vi "get_test_log_files.vi"(8 "error in (no error)":errorcluster, 11 "params in":T1) -> (0 "error out":errorcluster, 3 "Data":T2)   [LabVIEW 2015]
doc: "This vi does the following tasks: \n1.- Create the Test Log folder and subfolders, \n2.- Get the timeout values from config file, \n3.- Get the endpoint address from config file,\n4.- Get the file extension to search (i.e *json) from config file.,\n5.- Get holding time from config file."
uses:
  Type Definitions/get_test_log_files_data.ctl
  <vilib>/Utility/error.llb/Error Cluster From Error Code.vi
  <vilib>/ErrorRing/Error Ring.xnode
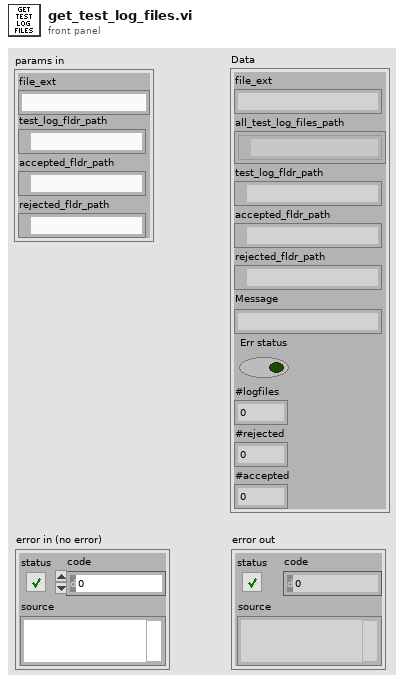
[diagram p1: front panel]
types:
  T1 = cluster{"file_ext":string, "test_log_fldr_path":path, "accepted_fldr_path":path, "rejected_fldr_path":path}
  T2 = typedef "get_test_log_files_data.ctl" = cluster{"file_ext":string, "all_test_log_files_path":path[], "test_log_fldr_path":path, "accepted_fldr_path":path, "rejected_fldr_path":path, "Message":string, "Err status":bool, "#logfiles":i32, "#rejected":i32, "#accepted":i32}
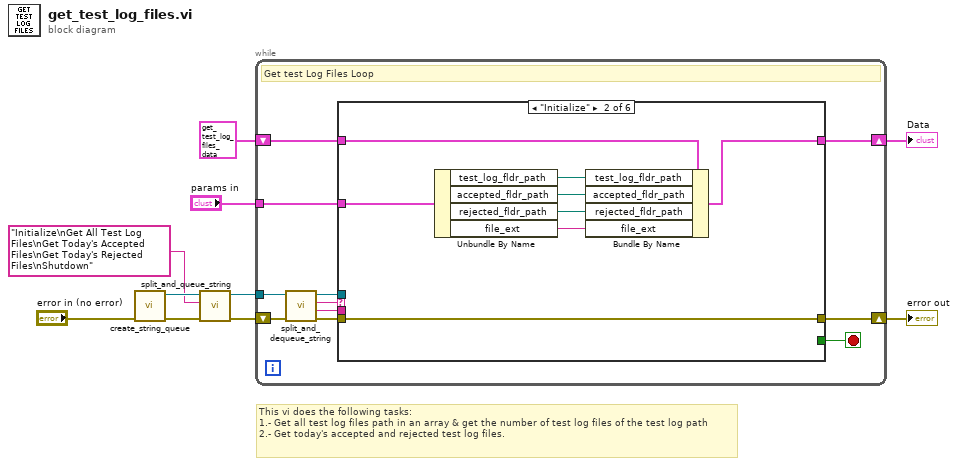
[diagram p0: block diagram]
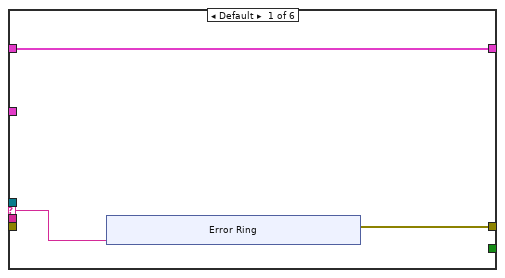
[diagram p2: hidden frame]
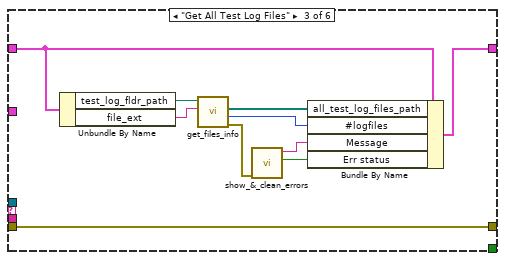
[diagram p3: hidden frame]
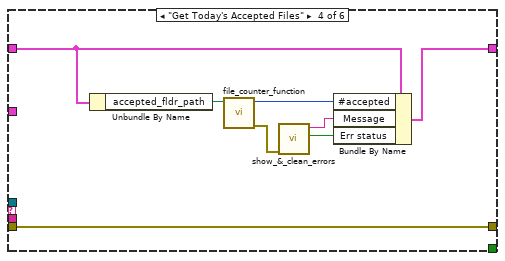
[diagram p4: hidden frame]
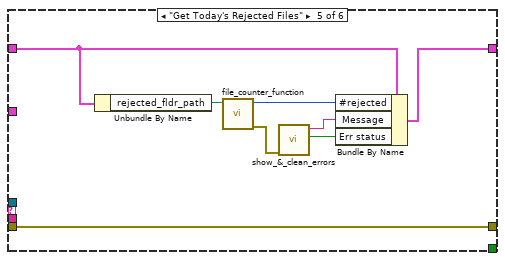
[diagram p5: hidden frame]
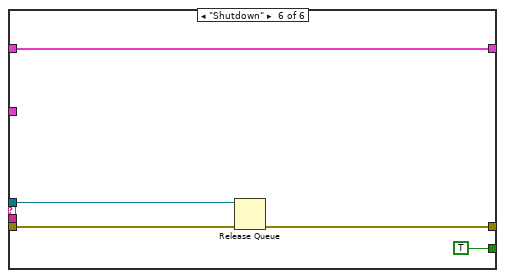
[diagram p6: hidden frame]
diagram:
  # "This vi does the following tasks:\n1.- Get all test log files path in an array & get the number of test log files of the test log path\n2.- Get today's accepted and rejected test log files."
  n1 = call "create_string_queue.vi"("error in (no error)"="error in (no error)") -> ("error out"=w9:errorcluster, "Queue out"=w10:refnum<queue>)  [unwired: 9 in]
  n2 = call "split_and_queue_string.vi"("error in (no error)"=w9, "list state:argument"="Initialize\nGet All Test Log Files\nGet Today's Accepted Files\nGet Today's Rejected Files\nShutdown", "Queue in"=w10) -> ("error out"=w8:errorcluster, "Queue out"=w7:refnum<queue>)  [unwired: 7 in]
  n3 = while {
    shift-right: [w19] -> w5
    shift-left: w8 -> [w21]
    tunnel: w7 -> [w17]
    shift-right: [w13] -> w2
    shift-left: T2 {"file_ext"="", "all_test_log_files_path"=[], "test_log_fldr_path"=path "", "accepted_fldr_path"=path "", "rejected_fldr_path"=path "", "Message"="", "Err status"=FALSE, "#logfiles"=0, "#rejected"=0, "#accepted"=0} ("Data") -> [w14]
    tunnel: "params in" -> [w11]
    stop <- w18 stop-if-true
    # "Get test Log Files Loop"
    n4 = call "split_and_dequeue_string.vi"("error in (no error)"=w21, "Queue in"=w17) -> ("error out"=w20:errorcluster, "argument"=w15:string, "state"=w16:string, "Queue out"=w12:refnum<queue>)  [unwired: 6 in]
    n5 = case shown="\"Initialize\"" w16 {
      selector: w16 -> [w23 _ _ _ _ _]
      tunnel: w20 -> [_ w39 w49 w57 w65 w69]
      tunnel: [w22 w39 w49 w57 w65 w67] -> w19
      tunnel: [_ _ _ _ _ TRUE] -> w18
      tunnel: w12 -> [_ _ _ _ _ w68]
      tunnel: w15 -> [_ _ _ _ _ _]
      tunnel: w14 -> [w24 w38 w41 w51 w59 w66]
      tunnel: [w24 w37 w40 w50 w58 w66] -> w13
      tunnel: w11 -> [_ w36 _ _ _ _]
      frame Default {
        n6 = xnode "Error Ring"("parameter 0"=w23) -> ("error out"=w22:errorcluster)
      }
      frame "Initialize" {
        n7 = Unbundle By Name(w36) -> ("test_log_fldr_path"=w34:path, "accepted_fldr_path"=w33:path, "rejected_fldr_path"=w32:path, "file_ext"=w35:string)
        n8 = Bundle By Name(cluster=w38, "test_log_fldr_path"=w34, "accepted_fldr_path"=w33, "rejected_fldr_path"=w32, "file_ext"=w35) -> (w37:T2)
      }
      frame "Get All Test Log Files" {
        n9 = Unbundle By Name(w41) -> ("test_log_fldr_path"=w47:path, "file_ext"=w48:string)
        n10 = call "get_files_info.vi"("file extension"=w48, "test_log_base_path"=w47) -> ("error out"=w42:errorcluster, "logfiles#"=w44:i32, "All files in folder"=w43:path[])  [unwired: 6 in, 1 out]
        n11 = call "show_&_clean_errors.vi"("error in (no error)"=w42) -> ("status"=w46:bool, "message out"=w45:string)  [unwired: 7 in, 2 out]
        n12 = Bundle By Name(cluster=w41, "all_test_log_files_path"=w43, "#logfiles"=w44, "Message"=w45, "Err status"=w46) -> (w40:T2)
      }
      frame "Get Today's Accepted Files" {
        n13 = Unbundle By Name(w51) -> ("accepted_fldr_path"=w54:path)
        n14 = call "file_counter_function.vi"("files_folder_path"=w54) -> ("error out"=w56:errorcluster, "#files_found"=w55:i32)  [unwired: 8 in, 1 out]
        n15 = call "show_&_clean_errors.vi"("error in (no error)"=w56) -> ("status"=w52:bool, "message out"=w53:string)  [unwired: 7 in, 2 out]
        n16 = Bundle By Name(cluster=w51, "#accepted"=w55, "Message"=w53, "Err status"=w52) -> (w50:T2)
      }
      frame "Get Today's Rejected Files" {
        n17 = Unbundle By Name(w59) -> ("rejected_fldr_path"=w62:path)
        n18 = call "file_counter_function.vi"("files_folder_path"=w62) -> ("error out"=w64:errorcluster, "#files_found"=w63:i32)  [unwired: 8 in, 1 out]
        n19 = call "show_&_clean_errors.vi"("error in (no error)"=w64) -> ("status"=w60:bool, "message out"=w61:string)  [unwired: 7 in, 2 out]
        n20 = Bundle By Name(cluster=w59, "#rejected"=w63, "Message"=w61, "Err status"=w60) -> (w58:T2)
      }
      frame "Shutdown" {
        n21 = Release Queue(queue=w68, error in (no error)=w69) -> (error out=w67:errorcluster)  [unwired: 1 in, 2 out]
      }
    }
  }
  "error out" <- w5
  "Data" <- w2
